vi "Update Test Result.vi"(6 "Data":string, 7 "Command":T1, 8 "error in (no error)":errorcluster, 9 "Table Index":i32=2, 10 "Test ID Index":i32, 11 "Test Result":refnum<vi>) -> (0 "error out":errorcluster)   [LabVIEW 2021, in "User Interface.lvlib"]
uses:
  User Interface.lvlib
  Test Status Command.ctl
  <vilib>/Utility/miscctls.llb/LVRowAndColumnTypeDef.ctl
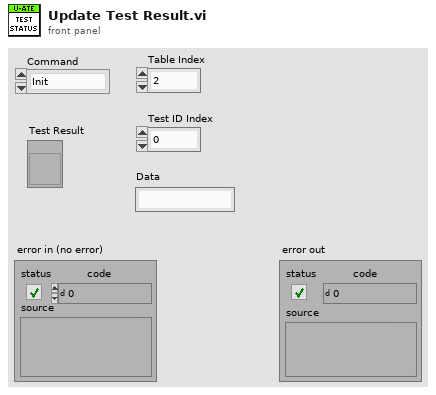
[diagram p1: front panel]
types:
  T1 = typedef "User Interface.lvlib/Test Status Command.ctl" = enum16{"Init", "Test Status"}
  T2 = typedef "LVRowAndColumnTypeDef.ctl" = cluster{"Row":i32, "Column":i32}
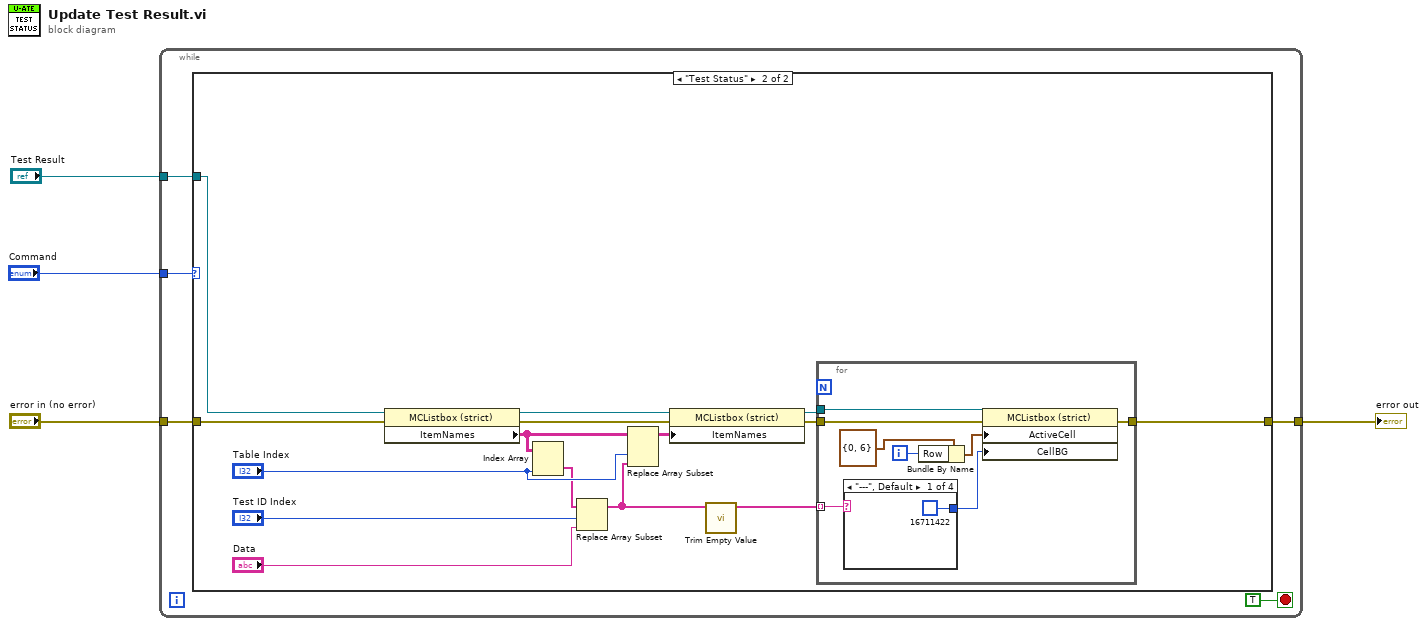
[diagram p0: block diagram]
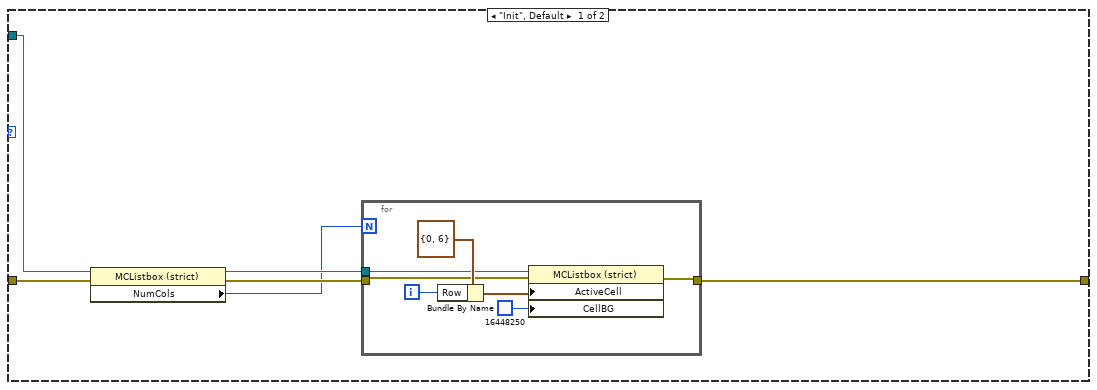
[diagram p2: hidden frame]
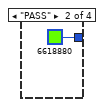
[diagram p3: hidden frame]
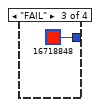
[diagram p4: hidden frame]
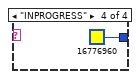
[diagram p5: hidden frame]
diagram:
  n1 = while {
    tunnel: "error in (no error)" -> [w8]
    tunnel: "Command" -> [w7]
    tunnel: "Test Result" -> [w6]
    tunnel: [w5] -> w1
    stop <- TRUE stop-if-true
    n2 = case shown="\"Test Status\"" w7 {
      tunnel: w8 -> [w14 w26]
      tunnel: w6 -> [w15 w24]
      tunnel: [w12 w25] -> w5
      frame "Init", Default {
        n3 = property class="MCListbox (strict)"(reference=w15, error in=w14) -> (reference out=w11:refnum<vi>, error out=w13:errorcluster, "NumCols"=w10:u32)
        n4 = for {
          N: w10 -> [_]
          tunnel: [w17] -> w12
          tunnel: w13 -> [w20]
          tunnel: w11 -> [w18]
          i -> [w21]
          n5 = Bundle By Name(cluster=T2 {"Row"=0, "Column"=6} ("Active Cell:Active Cell"), "Row"=w21) -> (w19:T2)
          n6 = property class="MCListbox (strict)"(reference=w18, error in=w20, "ActiveCell"=w19, "CellBG"=u32 16448250) -> (error out=w17:errorcluster)  [unwired: 1 out]
        }
      }
      frame "Test Status" {
        n7 = property class="MCListbox (strict)"(reference=w24, error in=w26) -> (reference out=w31:refnum<vi>, error out=w32:errorcluster, "ItemNames"=w33:string[][])
        n8 = Index Array(array=w33, index (col)="Table Index") -> (element=w34:string[])  [unwired: 1 in]
        n9 = Replace Array Subset(array=w34, new element="Data", index="Test ID Index") -> (w28:string[])
        n10 = Replace Array Subset(array=w33, new element=w28, index (col)="Table Index") -> (w27:string[][])  [unwired: 1 in]
        n11 = property class="MCListbox (strict)"(reference=w31, error in=w32, "ItemNames"=w27) -> (reference out=w29:refnum<vi>, error out=w30:errorcluster)
        n12 = call "Trim Empty Value.vi"("Data In"=w28) -> ("Data Out"=w23:string[])  [unwired: 10 in]
        n13 = for {
          tunnel: w30 -> [w43]
          tunnel: w29 -> [w44]
          tunnel: w23 -> [w45] mode=indexing
          tunnel: [w38] -> w25
          i -> [w41]
          n14 = case shown="\"---\", Default" w45 {
            tunnel: [u32 16711422 u32 6618880 u32 16718848 u32 16776960] -> w39
            frame "---", Default {
            }
            frame "PASS" {
            }
            frame "FAIL" {
            }
            frame "INPROGRESS" {
            }
          }
          n15 = Bundle By Name(cluster=T2 {"Row"=0, "Column"=6} ("Active Cell:Active Cell"), "Row"=w41) -> (w40:T2)
          n16 = property class="MCListbox (strict)"(reference=w44, error in=w43, "ActiveCell"=w40, "CellBG"=w39) -> (error out=w38:errorcluster)  [unwired: 1 out]
        }
      }
    }
  }
  "error out" <- w1
